vi "CC Observation Object to Script Command.vi"(8 "error in (no error)":errorcluster, 9 "Offsets":T3, 10 "RA and DEC String":cluster{"RA":string, "DEC":string}={"RA"="HH:MM:SS.nnn", "DEC"="DEG:arcmin:arcsec.nn"} caption="RA and DEC", 11 "Object.Name":string) -> (0 "error out":errorcluster, 2 "Object Name out":string, 3 "Define Object Step":T1={"Action"=enum."Acquire Images", "Data"=variant})   [LabVIEW 2021]
uses:
  Telescope/CC cluster Telescope Offsets.ctl
  typedefs/CC Script Step.ctl
  typedefs/CC enum Script Action.ctl
  typedefs/CC cluster Object.ctl
  typedefs/CC cluster sidereal rate.ctl
  typedefs/CC cluster RA and DEC.ctl
  typedefs/cc cluster muRA muDEC.ctl
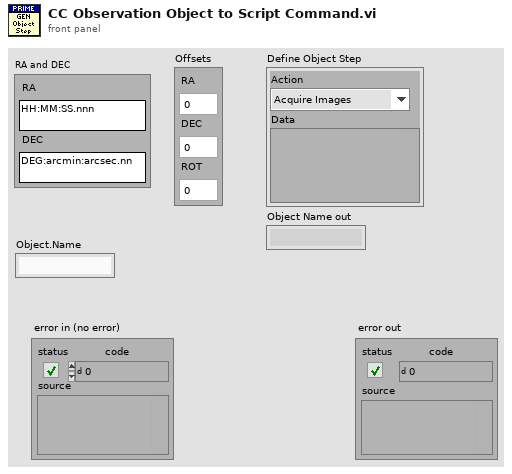
[diagram p1: front panel]
types:
  T1 = typedef "CC Script Step.ctl" = cluster{"Action":T2, "Data":variant}
  T2 = typedef "CC enum Script Action.ctl" = enum16{"Noop", "Define Object", "Define Exposure", "Define Dithering", "Acquire Images", "Set Filter Wheel", "Telescope Home", "Telescope Move", "Telescope RA DEC", "Focus Move Relative", "Focus Move Absolute", "Focus Set Home", "Macro", "Pause", "Ask User", "Define Random Dither"}
  T3 = typedef "CC cluster Telescope Offsets.ctl" = cluster{"RA":dbl, "DEC":dbl, "ROT":dbl}
  T4 = typedef "CC cluster Object.ctl" = cluster{"Object":cluster{"Name":string}, "Sidereal Rate":T5, "RA and DEC":T6, "muRA muDEC Epoch":T7, "Offsets":T3}
  T5 = typedef "CC cluster sidereal rate.ctl" = cluster{"dRA":dbl, "dDEC":dbl}
  T6 = typedef "CC cluster RA and DEC.ctl" = cluster{"RA":dbl, "DEC":dbl}
  T7 = typedef "cc cluster muRA muDEC.ctl" = cluster{"muRA":dbl, "muDEC":dbl, "Epoch":dbl}
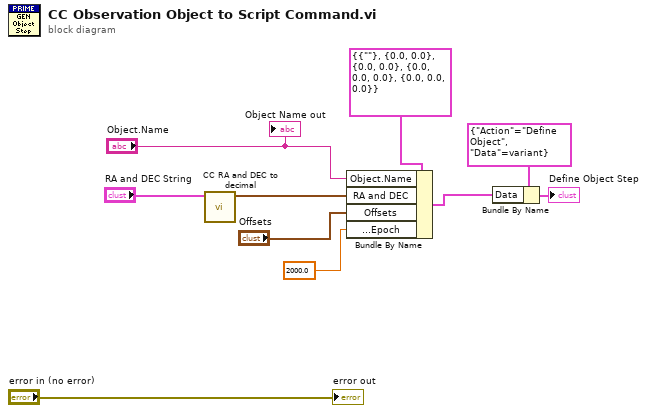
[diagram p0: block diagram]
diagram:
  n1 = call "CC RA and DEC to decimal.vi"("RA and DEC String"="RA and DEC String") -> ("RA and DEC"=w3:T6)  [unwired: 9 in, 1 out]
  n2 = Bundle By Name(cluster=T4 {"Object"={"Name"=""}, "Sidereal Rate"={"dRA"=0.0, "dDEC"=0.0}, "RA and DEC"={"RA"=0.0, "DEC"=0.0}, "muRA muDEC Epoch"={"muRA"=0.0, "muDEC"=0.0, "Epoch"=0.0}, "Offsets"={"RA"=0.0, "DEC"=0.0, "ROT"=0.0}} ("Object"), "Object.Name"="Object.Name", "RA and DEC"=w3, "Offsets"="Offsets", "muRA muDEC Epoch.Epoch"=2000.0) -> (w7:T4)
  n3 = Bundle By Name(cluster=T1 {"Action"=enum."Define Object", "Data"=variant} ("Cluster"), "Data"=w7) -> (→"Define Object Step":T1)
  "error out" <- "error in (no error)"
  "Object Name out" <- "Object.Name"
